vi "WSVCAP SHL FPGA LL Procedure RFFE - Send SSC.vi"(0 "Procedure Step":T1, 1 "Wait Ticks Remaining":u32, 5 "Wait Ticks":u32, 11 "error in (no error)":errorcluster, 13 "Socket Mask":u64) -> (3 "Wait Ticks Remaining Out":u32, 4 "Procedure Step Out":T1, 10 "Finished":bool, 15 "error out":errorcluster)   [LabVIEW 2017]
uses:
  Type Defs/WSVCAP SHL Procedure Step Enum.ctl
  Type Defs/WSVCAP SHL RFFE Write Line Enum.ctl
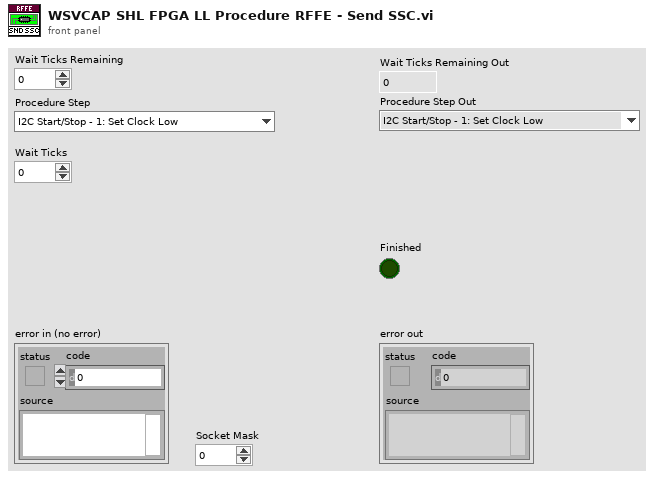
[diagram p1: front panel]
types:
  T1 = typedef "WSVCAP SHL Procedure Step Enum.ctl" = enum16{"I2C Start/Stop - 1: Set Clock Low", "I2C Start/Stop - 2: Wait", "I2C Start/Stop - 3: Set Data I", "I2C Start/Stop - 4: Wait", "I2C Start/Stop - 5: Set Clock High", "I2C Start/Stop - 6: Wait", "I2C Start/Stop - 7: Set Data II", "I2C Start/Stop - 8: Wait", "I2C Start/Stop - 9: Set Clock Low", "I2C Start/Stop - 10: Wait", "I2C Read ACK - 1: Set Clock High", "I2C Read ACK - 2: Wait", "I2C Read ACK - 3: Read ACK Bit", "I2C Read ACK - 4: Wait", "I2C Read ACK - 5: Set Clock Low", "I2C Read ACK - 6: Wait", "I2C Write ACK - 1: Write ACK Bit", "I2C Write ACK - 2: Wait", "I2C Write ACK - 3: Set Clock High", "I2C Write ACK - 4: Wait", "I2C Write ACK - 5: Set Clock Low", "I2C Write ACK - 6: Wait", "I2C Write ACK - 7: Set Data Low", "I2C Send Add - 1: Reset Bits Remaining", "I2C Send Add - 2: Set Data Bit", "I2C Send Add - 3: Wait", "I2C Send Add - 4: Set Clock High", "I2C Send Add - 5: Wait", "I2C Send Add - 6: Set Clock Low", "I2C Send Add - 7: Wait", "I2C Send Add - 8: Check Bits Remaining", "I2C Send Data - 1: Reset Bits Remaining", "I2C Send Data - 2: Load Write Bit from FIFO", "I2C Send Data - 3: Set Data Bit", "I2C Send Data - 4: Wait", "I2C Send Data - 5: Set Clock High", "I2C Send Data - 6: Wait", "I2C Send Data - 7: Set Clock Low", "I2C Send Data - 8: Wait", "I2C Send Data - 9: Check Bits Remaining", "I2C Receive Data - 1: Reset Bits Remaining", "I2C Receive Data - 2: Wait", "I2C Receive Data - 3: Set Clock High", "I2C Receive Data - 4: Wait", "I2C Receive Data - 5: Read Data Bit", "I2C Receive Data - 6: Wait", "I2C Receive Data - 7: Set Clock Low", "I2C Receive Data - 8: Wait", "I2C Receive Data - 9: Check Bits Remaining", "RFFE Send SSC - 1:Set Low", "RFFE Send SSC - 2:Wait", "RFFE Send SSC - 3:Set SDA High", "RFFE Send SSC - 4:Wait", "RFFE Send SSC - 5:Set SDA Low", "RFFE Send SSC - 6:Wait", "RFFE Send Data - 1:Set SCL High", "RFFE Send Data - 2:Wait", "RFFE Send Data - 3:Set SCL Low", "RFFE Send Data - 4:Wait", "RFFE Send Data - 5:Set SCL High (P)", "RFFE Send Data - 6:Wait", "RFFE Send Data - 7:Set SCL Low (P)", "RFFE Send Data - 8:Wait", "RFFE Send Data - 9:Set SCL High (BP)", "RFFE Send Data - 10:Wait", "RFFE Send Data - 11:Set SCL Low (BP)", "RFFE Send Data - 12:Wait", "RFFE Receive Data - 1:Set SCL High", "RFFE Receive Data - 2:Wait", "RFFE Receive Data - 3:Set SCL Low", "RFFE Receive Data - 4:Wait", "RFFE Receive Data - 5:Set SCL High (BP)", "RFFE Receive Data - 6:Wait", "RFFE Receive Data - 7:Set SCL Low (BP)", "RFFE Receive Data - 8:Wait", "RFFE Wait CMD Delay - 1:Wait", "RFFE Clear Lines - 1:Clear", "SRL Write Data - 1:Set SYNC Low", "SRL Write Data - 2:Set SCLK High", "SRL Write Data - 3:Wait", "SRL Write Data - 4:Set SCLK Low", "SRL Write Data - 5:Wait", "SRL Write Data - 6:Set SYNC High", "SRL Wait CMD Delay - 1:Wait", "SRL Clear Lines - 1:Clear"}
  T2 = typedef "WSVCAP SHL RFFE Write Line Enum.ctl" = enum16{"SDAA", "SCLK"}
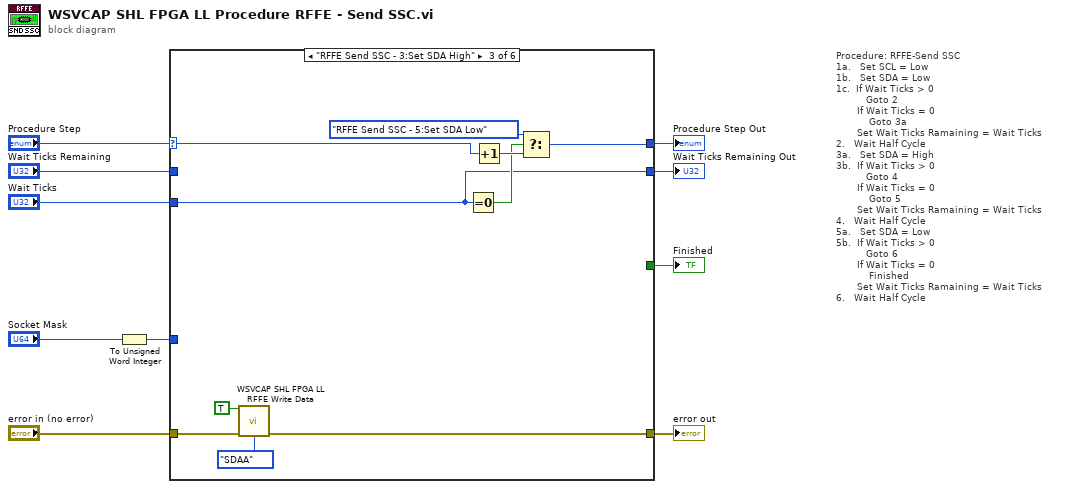
[diagram p0: block diagram]
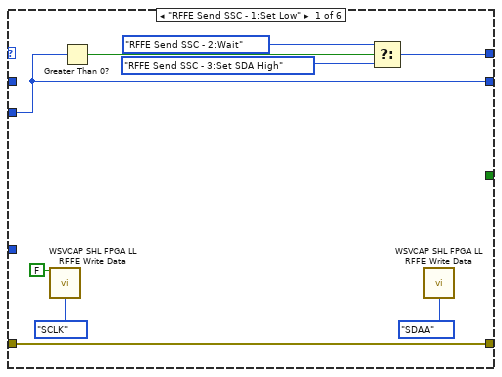
[diagram p2: hidden frame]
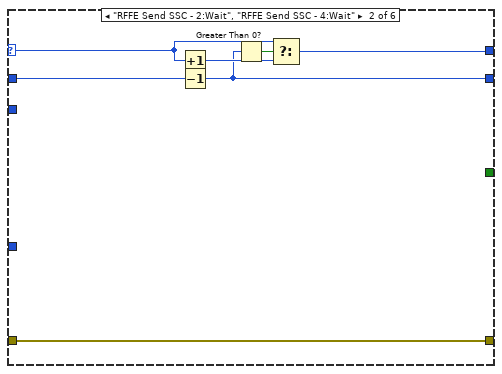
[diagram p3: hidden frame]
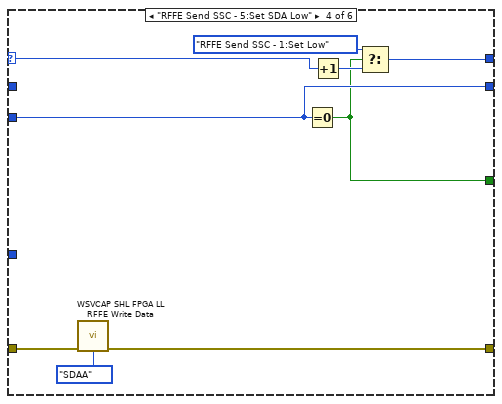
[diagram p4: hidden frame]
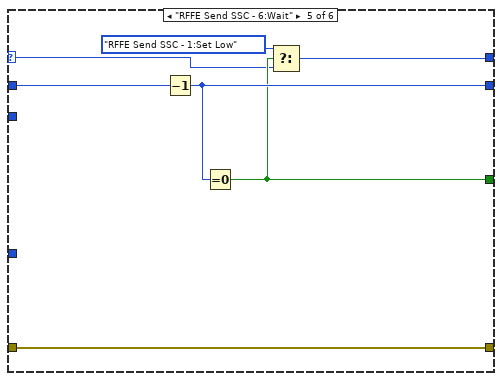
[diagram p5: hidden frame]
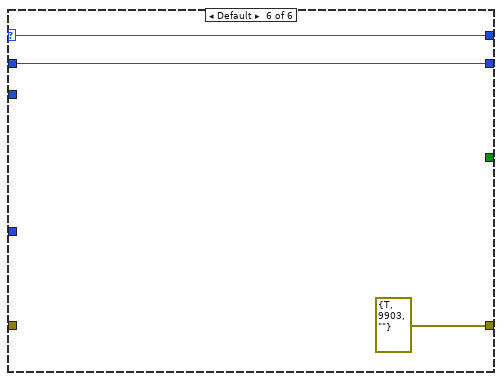
[diagram p6: hidden frame]
diagram:
  # "Procedure: RFFE-Send SSC\n1a.   Set SCL = Low\n1b.   Set SDA = Low\n1c.  If Wait Ticks > 0\n          Goto 2\n       If Wait Ticks = 0 \n           Goto 3a\n       Set Wait Ticks Ramaining = Wait Ticks\n2.   Wait Half Cycle\n3a.   Set SDA = High\n3b.  If Wait Ticks > 0\n          Goto 4\n       If Wait Ticks = 0 \n           Goto 5\n       Set Wait Ticks Ramaining = Wait Ticks\n4.   Wait Half Cycle\n5a.   Set SDA = Low\n5b.  If Wait Ticks > 0\n          Goto 6\n       If Wait Ticks = 0 \n           Finished\n       Set Wait Ticks Ramaining = Wait Ticks\n6.   Wait Half Cycle"
  n1 = To Unsigned Word Integer(number="Socket Mask") -> (unsigned 16bit integer=w7:u16)
  n2 = case shown="\"RFFE Send SSC - 3:Set SDA High\"" "Procedure Step" {
    selector: "Procedure Step" -> [_ w24 w36 w45 w46 w54]
    tunnel: [w17 w26 w33 w42 w52 errorcluster {"status"=TRUE, "code"=9903, "source"=""} ("error IO")] -> w9
    tunnel: "error in (no error)" -> [w17 w26 w34 w43 w52 _]
    tunnel: "Wait Ticks Remaining" -> [_ w22 _ _ w51 w53]
    tunnel: "Wait Ticks" -> [w13 _ w29 w39 _ _]
    tunnel: [_ _ _ w37 w48 _] -> w8
    tunnel: w7 -> [_ _ _ _ _ _]
    tunnel: [w14 w21 w30 w40 w50 w54] -> w2
    tunnel: [w13 w20 w29 w39 w49 w53] -> w1
    frame "RFFE Send SSC - 1:Set Low" {
      n3 = call "WSVCAP SHL FPGA LL RFFE Write Data.vi"("Bit In"=FALSE, "Line"=WSVCAP_SHL_RFFE_Write_Line_Enum."SCLK") -> ()  [unwired: 13 in, 1 out]
      n4 = Greater Than 0?(x=w13) -> (x > 0?=w18:bool)
      n5 = Select(t=WSVCAP_SHL_Procedure_Step_Enum."RFFE Send SSC - 2:Wait" ("Procedure Step"), s=w18, f=WSVCAP_SHL_Procedure_Step_Enum."RFFE Send SSC - 3:Set SDA High" ("Procedure Step")) -> (s? t:f=w14:T1)
      n6 = call "WSVCAP SHL FPGA LL RFFE Write Data.vi"("Line"=WSVCAP_SHL_RFFE_Write_Line_Enum."SDAA") -> ()  [unwired: 14 in, 1 out]
    }
    frame "RFFE Send SSC - 2:Wait", "RFFE Send SSC - 4:Wait" {
      n7 = Increment(x=w24) -> (x+1=w23:T1)
      n8 = Decrement(x=w22) -> (x-1=w20:u32)
      n9 = Greater Than 0?(x=w20) -> (x > 0?=w25:bool)
      n10 = Select(t=w24, s=w25, f=w23) -> (s? t:f=w21:T1)
    }
    frame "RFFE Send SSC - 3:Set SDA High" {
      n11 = call "WSVCAP SHL FPGA LL RFFE Write Data.vi"("Bit In"=TRUE, "error in (no error)"=w34, "Line"=WSVCAP_SHL_RFFE_Write_Line_Enum."SDAA") -> ("error out"=w33:errorcluster)  [unwired: 12 in]
      n12 = Equal To 0?(x=w29) -> (x = 0?=w32:bool)
      n13 = Increment(x=w36) -> (x+1=w35:T1)
      n14 = Select(t=WSVCAP_SHL_Procedure_Step_Enum."RFFE Send SSC - 5:Set SDA Low" ("Procedure Step"), s=w32, f=w35) -> (s? t:f=w30:T1)
    }
    frame "RFFE Send SSC - 5:Set SDA Low" {
      n15 = call "WSVCAP SHL FPGA LL RFFE Write Data.vi"("error in (no error)"=w43, "Line"=WSVCAP_SHL_RFFE_Write_Line_Enum."SDAA") -> ("error out"=w42:errorcluster)  [unwired: 13 in]
      n16 = Equal To 0?(x=w39) -> (x = 0?=w37:bool)
      n17 = Increment(x=w45) -> (x+1=w44:T1)
      n18 = Select(t=WSVCAP_SHL_Procedure_Step_Enum."RFFE Send SSC - 1:Set Low" ("Procedure Step"), s=w37, f=w44) -> (s? t:f=w40:T1)
    }
    frame "RFFE Send SSC - 6:Wait" {
      n19 = Decrement(x=w51) -> (x-1=w49:u32)
      n20 = Equal To 0?(x=w49) -> (x = 0?=w48:bool)
      n21 = Select(t=WSVCAP_SHL_Procedure_Step_Enum."RFFE Send SSC - 1:Set Low" ("f"), s=w48, f=w46) -> (s? t:f=w50:T1)
    }
    frame Default {
    }
  }
  "error out" <- w9
  "Finished" <- w8
  "Procedure Step Out" <- w2
  "Wait Ticks Remaining Out" <- w1
